vi "Send Telemetry Descriptor Event.vi"(8 "error in":errorcluster, 10 "Telemetry_Descriptors":variant, 11 "Engine in":refnum<class "Engine.lvclass">) -> (0 "error out":errorcluster, 3 "Engine out":refnum<class "Engine.lvclass">)   [LabVIEW 2019, in "Engine.lvlib" / "Engine.lvclass"]
doc: "This routine transmits an telemetry descriptor event. Ancestor classes are responsible for determining whether or not they are the legal target and if the variant is well formed."
uses:
  Project/Engine.lvclass
  Project/Engine.lvclass/Engine.ctl
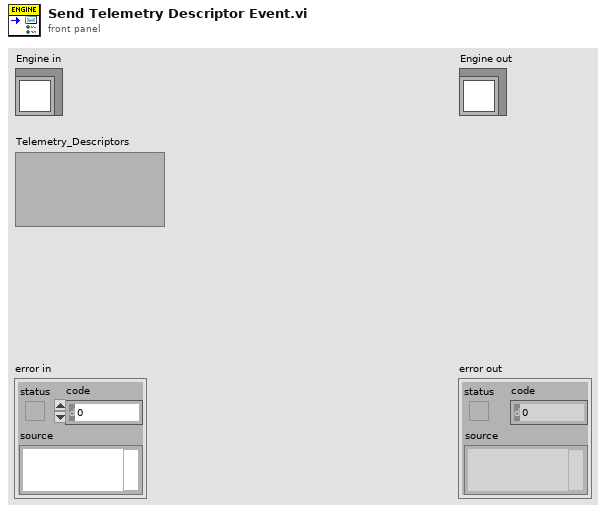
[diagram p1: front panel]
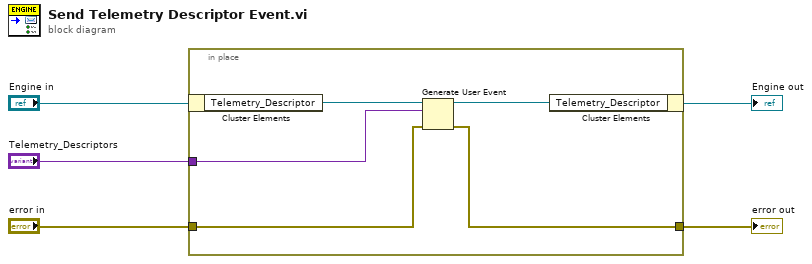
[diagram p0: block diagram]
diagram:
  n1 = in-place {
    in-place-border: "error in" -> [w8]
    in-place-border: [w7] -> w2
    in-place-border: "Telemetry_Descriptors" -> [w6]
    n2 = in-place-cluster #1("Engine in") -> ("Telemetry_Descriptor"=w10:refnum<user-event>)
    n3 = Generate User Event(user event=w10, event data cluster=w6, error in=w8) -> (user event out=w9:refnum<user-event>, error out=w7:errorcluster)  [unwired: 1 in]
    n4 = in-place-cluster #1("Telemetry_Descriptor"=w9) -> (→"Engine out":refnum<class "Engine.lvclass">)
  }
  "error out" <- w2
